vi "BondingPicture.vi"(9 "Z-Position":dbl format="%#_13g") -> (1 "new picture":picture)   [LabVIEW 2023]
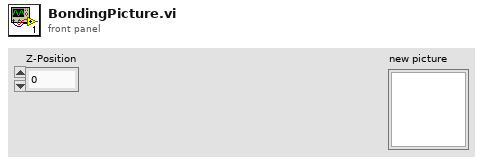
[diagram p1: front panel]
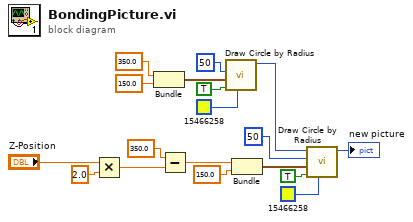
[diagram p0: block diagram]
diagram:
  n1 = Multiply(x="Z-Position", y=2.0) -> (x*y=w3:dbl)
  n2 = Bundle(350.0, 150.0) -> (w15:cluster{dbl, dbl})  [unwired: 1 in]
  n3 = Subtract(x=350.0, y=w3) -> (x-y=w4:dbl)
  n4 = call <vilib>:"Draw Circle by Radius.vi"("color(black)"=u32 15466258, "fill?(F)"=TRUE, "pixel center"=w15, "radius"=i16 50) -> ("new picture"=w7:picture)  [unwired: 7 in]
  n5 = Bundle(w4, 150.0) -> (w11:cluster{dbl, dbl})  [unwired: 1 in]
  n6 = call <vilib>:"Draw Circle by Radius.vi"("color(black)"=u32 15466258, "fill?(F)"=TRUE, "pixel center"=w11, "radius"=i16 50, "picture"=w7) -> ("new picture"=→"new picture":picture)  [unwired: 6 in]
